vi "Test_Gui_Settings_With_Tabs.vi"() -> ()   [LabVIEW 2015]
uses:
  controls/GUI_Settings_Tabs.ctl
  controls/QMH_Pirenea_MessageCluster.ctl
panel:
  out "error out":errorcluster
  in  "error in (no error)":errorcluster
  in  "Stop":bool
  in  "Start":bool
  in  "Save":bool
  in  "Load":bool
  in  "Exit":bool
  in  "Settings":bool
  out "Commande onglets":enum32{"General", "Hardware", "Experiment"}(tab)
  out "PIL Status":string
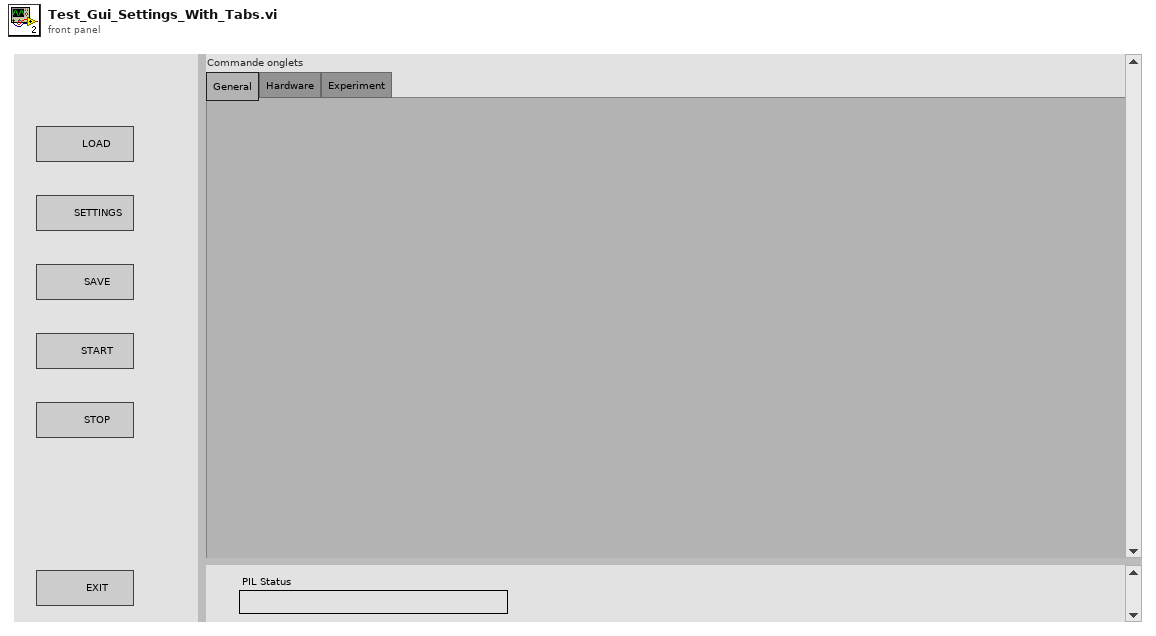
[diagram p1: front panel]
types:
  T1 = enum16{"Initialize", "Load", "Settings", "Save", "Start", "Stop", "Exit"}
  T2 = typedef "QMH_Pirenea_MessageCluster.ctl" = cluster{"Command":enum16{"Initialize", "Load", "Settings", "Save", "Start", "Stop", "Exit"}, "Data":variant}
  T3 = typedef "GUI_Settings_Tabs.ctl" = enum32{"General", "Hardware", "Experiment"}
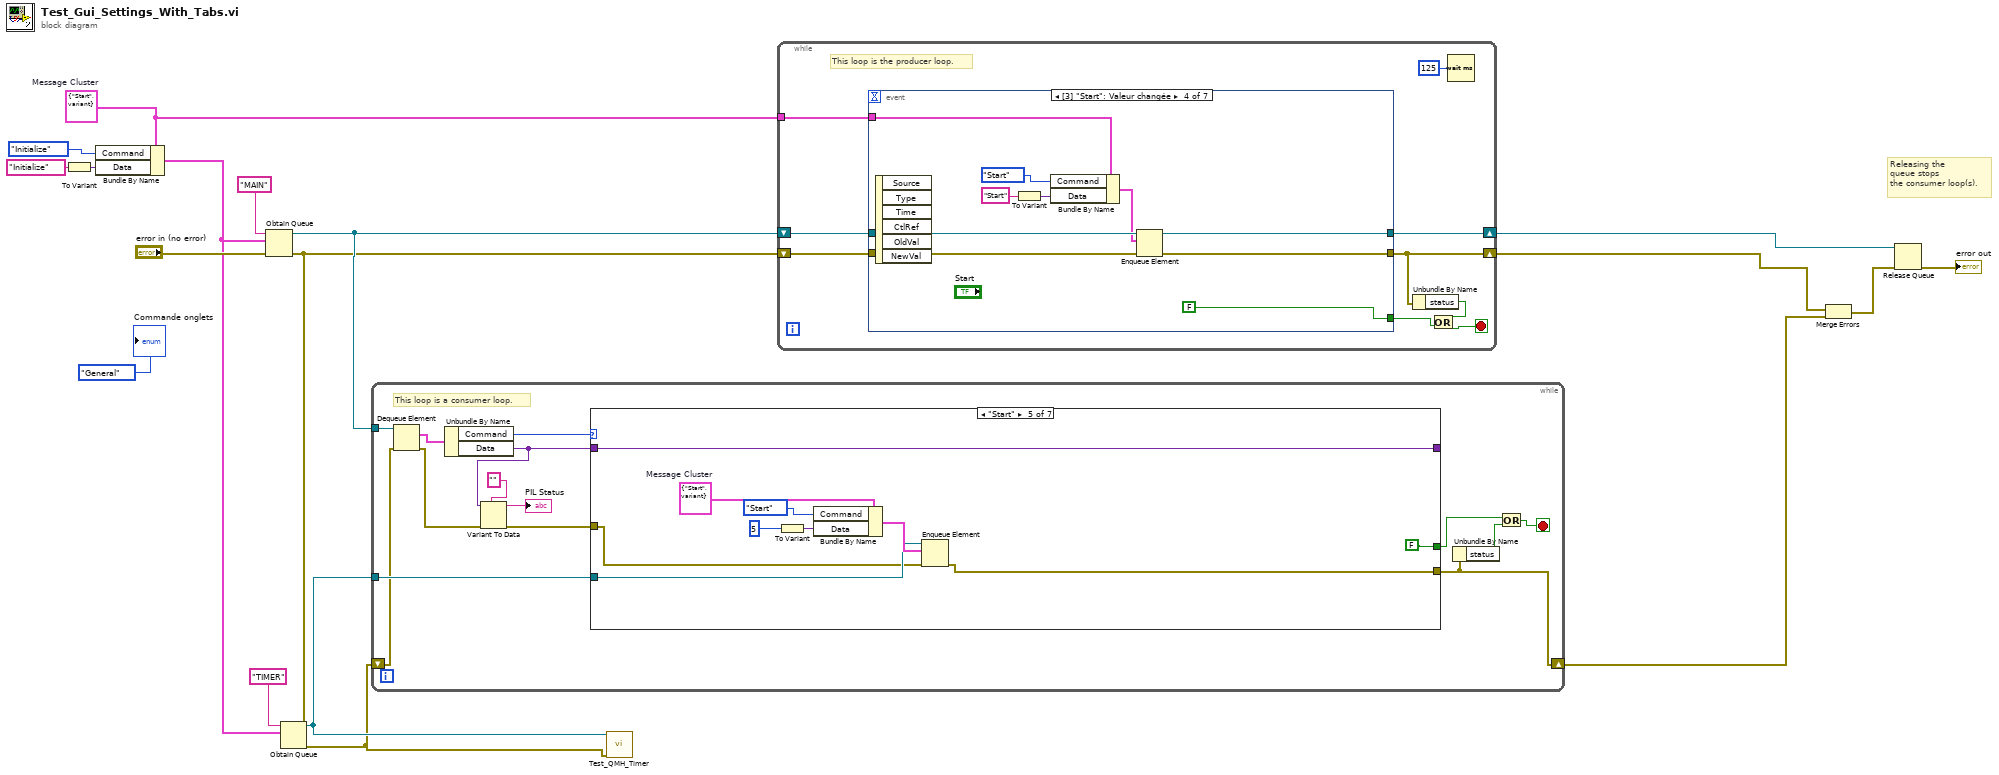
[diagram p0: block diagram]
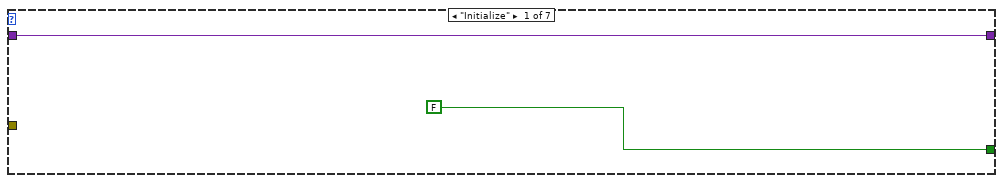
[diagram p2: hidden frame]
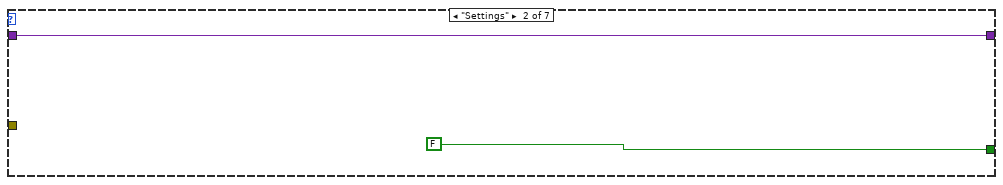
[diagram p3: hidden frame]
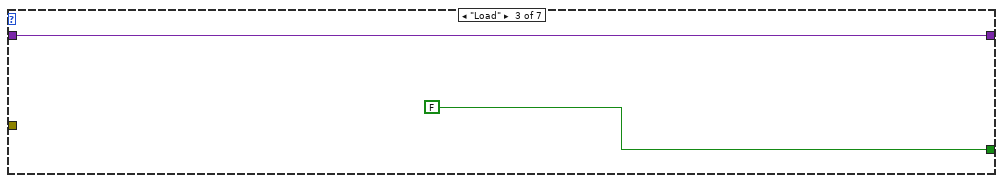
[diagram p4: hidden frame]
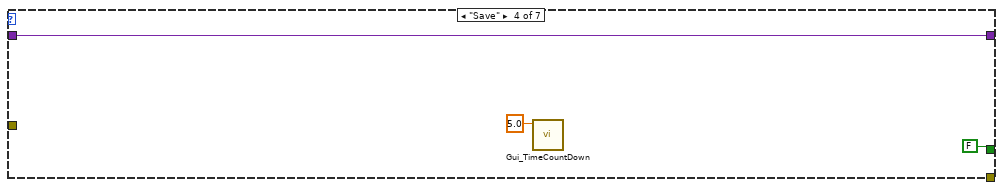
[diagram p5: hidden frame]
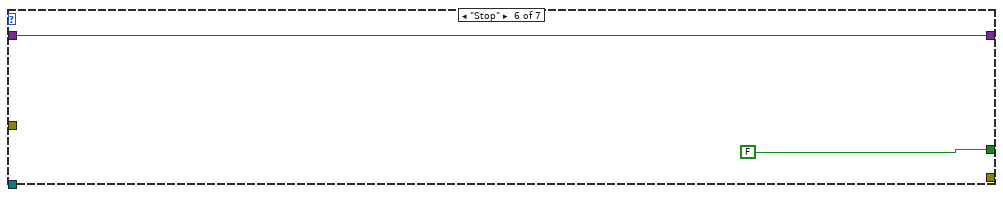
[diagram p6: hidden frame]
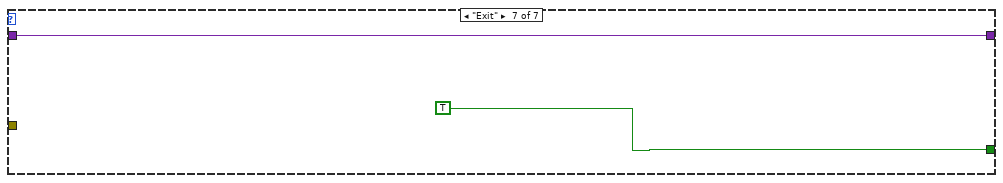
[diagram p7: hidden frame]
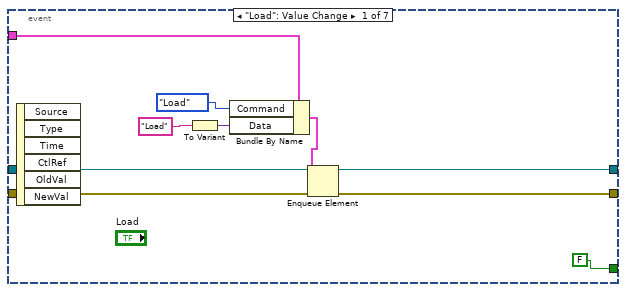
[diagram p8: hidden frame]
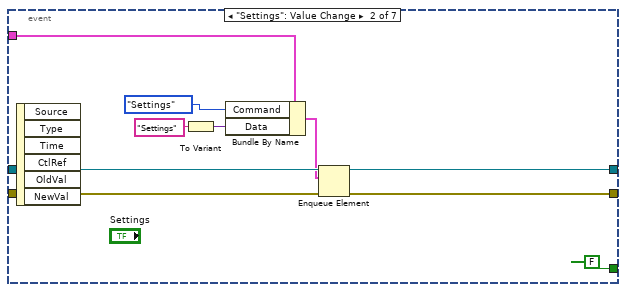
[diagram p9: hidden frame]
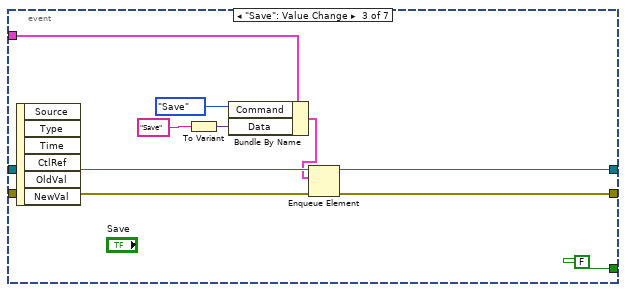
[diagram p10: hidden frame]
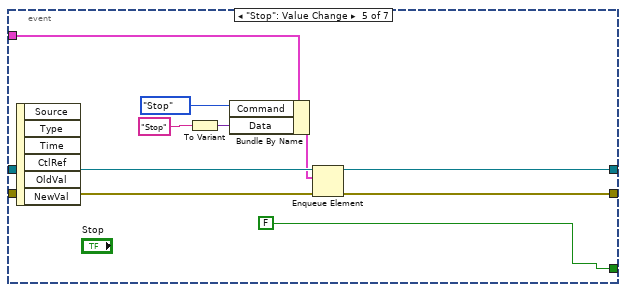
[diagram p11: hidden frame]
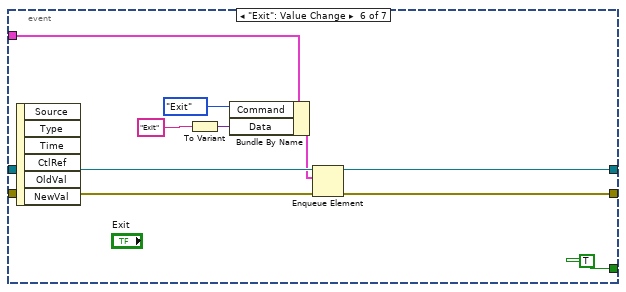
[diagram p12: hidden frame]
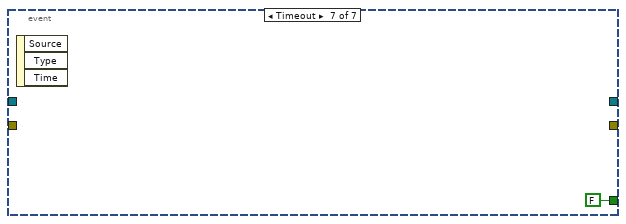
[diagram p13: hidden frame]
diagram:
  w9 = T2 {"Command"=enum."Start", "Data"=variant}  # Message Cluster
  # "Releasing the\nqueue stops\nthe consumer loop(s)."
  n1 = To Variant(anything="Initialize") -> (Variant=w10:variant)
  n2 = Bundle By Name(cluster=w9, "Command"=T1."Initialize", "Data"=w10) -> (w5:T2)
  n3 = Obtain Queue(name (unnamed)="MAIN" ("nom (aucun)"), element data type=w5, error in (no error)="error in (no error)") -> (queue out=w17:refnum<queue>, error out=w4:errorcluster)  [unwired: 2 in, 1 out]
  n4 = Obtain Queue(name (unnamed)="TIMER" ("nom (aucun)"), element data type=w5, error in (no error)=w4) -> (queue out=w2:refnum<queue>, error out=w1:errorcluster)  [unwired: 2 in, 1 out]
  n5 = while {
    tunnel: w17 -> [w31]
    tunnel: w2 -> [w21]
    shift-right: [w19] -> w3
    shift-left: w1 -> [w20]
    stop <- w25 stop-if-true
    # "This loop is a consumer loop."
    n6 = Dequeue Element(queue=w31, error in (no error)=w20) -> (element=w27:T2, error out=w28:errorcluster)  [unwired: 3 out]
    n7 = Unbundle By Name(w27) -> ("Command"=w23:T1, "Data"=w24:variant)
    n8 = Variant To Data(type="", Variant=w24) -> (data=→"PIL Status":string)  [unwired: 1 in, 1 out]
    n9 = case shown="\"Start\"" w23 {
      tunnel: [w32 w34 w36 w40 w49 w51 w53] -> _
      tunnel: [FALSE ("x") FALSE ("x") FALSE ("x") FALSE ("x") FALSE ("x") FALSE ("x") TRUE ("x")] -> w29
      tunnel: w24 -> [w32 w34 w36 w40 w49 w51 w53]
      tunnel: w28 -> [_ _ _ _ w42 _ _]
      tunnel: w21 -> [_ _ _ _ w45 _ _]
      tunnel: [_ _ _ _ w43 _ _] -> w19
      frame "Initialize" {
      }
      frame "Settings" {
      }
      frame "Load" {
      }
      frame "Save" {
        n10 = call "Gui_TimeCountDown.vi"("Seconds"=5.0) -> ()  [unwired: 11 in]
      }
      frame "Start" {
        w44 = T2 {"Command"=enum."Start", "Data"=variant}  # Message Cluster
        n11 = To Variant(anything=5) -> (Variant=w48:variant)
        n12 = Bundle By Name(cluster=w44, "Command"=T1."Start", "Data"=w48) -> (w46:T2)
        n13 = Enqueue Element(queue=w45, element=w46, error in (no error)=w42) -> (error out=w43:errorcluster)  [unwired: 3 out]
      }
      frame "Stop" {
      }
      frame "Exit" {
      }
    }
    n14 = Unbundle By Name(w19) -> ("status"=w30:bool)
    n15 = Or(x=w29, y=w30) -> (x .or. y?=w25:bool)
  }
  n16 = call "Test_QMH_Timer.vi"("error in (no error)"=w1, "Queue TIMER"=w2) -> ()  [unwired: 9 in, 1 out]
  n17 = while {
    shift-right: [w59] -> w12
    shift-left: w4 -> [w60]
    shift-right: [w58] -> w16
    shift-left: w17 -> [w61]
    tunnel: w9 -> [w56]
    stop <- w63 stop-if-true
    # "This loop is the producer loop."
    n18 = event shown="[3] \"Start\": Valeur changée" {
      selector: _ -> [_ _ _ _ _ _ _]
      dyn-events: _ -> [_ _ _ _ _ _ _]
      timeout: _ -> [_ _ _ _ _ _ _]
      tunnel: w61 -> [w73 w83 w93 w103 w113 w123 _]
      tunnel: w60 -> [w72 w82 w92 w102 w112 w122 _]
      tunnel: [w71 w81 w91 w101 w111 w121 _] -> w59
      tunnel: [w70 w80 w90 w100 w110 w120 _] -> w58
      tunnel: [FALSE ("Stop") FALSE ("Stop") FALSE ("Stop") FALSE ("Stop") FALSE ("Stop") TRUE ("Stop") FALSE ("Stop")] -> w57
      tunnel: w56 -> [w66 w76 w86 w96 w106 w116 _]
      event "Load": Value Change {
        n19 = event-data() -> ()  [unwired: 7 out]
        n20 = To Variant(anything="Load") -> (Variant=w68:variant)
        n21 = Bundle By Name(cluster=w66, "Command"=T1."Load", "Data"=w68) -> (w65:T2)
        n22 = Enqueue Element(queue=w73, element=w65, error in (no error)=w72) -> (queue out=w70:refnum<queue>, error out=w71:errorcluster)  [unwired: 2 out]
      }
      event "Settings": Value Change {
        n23 = event-data() -> ()  [unwired: 7 out]
        n24 = To Variant(anything="Settings") -> (Variant=w78:variant)
        n25 = Bundle By Name(cluster=w76, "Command"=T1."Settings", "Data"=w78) -> (w75:T2)
        n26 = Enqueue Element(queue=w83, element=w75, error in (no error)=w82) -> (queue out=w80:refnum<queue>, error out=w81:errorcluster)  [unwired: 2 out]
      }
      event "Save": Value Change {
        n27 = event-data() -> ()  [unwired: 7 out]
        n28 = To Variant(anything="Save") -> (Variant=w88:variant)
        n29 = Bundle By Name(cluster=w86, "Command"=T1."Save", "Data"=w88) -> (w85:T2)
        n30 = Enqueue Element(queue=w93, element=w85, error in (no error)=w92) -> (queue out=w90:refnum<queue>, error out=w91:errorcluster)  [unwired: 2 out]
      }
      event "Start": Value Change {
        n31 = event-data() -> ()  [unwired: 7 out]
        n32 = To Variant(anything="Start") -> (Variant=w97:variant)
        n33 = Bundle By Name(cluster=w96, "Command"=T1."Start", "Data"=w97) -> (w95:T2)
        n34 = Enqueue Element(queue=w103, element=w95, error in (no error)=w102) -> (queue out=w100:refnum<queue>, error out=w101:errorcluster)  [unwired: 2 out]
      }
      event "Stop": Value Change {
        n35 = event-data() -> ()  [unwired: 7 out]
        n36 = To Variant(anything="Stop") -> (Variant=w108:variant)
        n37 = Bundle By Name(cluster=w106, "Command"=T1."Stop", "Data"=w108) -> (w105:T2)
        n38 = Enqueue Element(queue=w113, element=w105, error in (no error)=w112) -> (queue out=w110:refnum<queue>, error out=w111:errorcluster)  [unwired: 2 out]
      }
      event "Exit": Value Change {
        n39 = event-data() -> ()  [unwired: 7 out]
        n40 = To Variant(anything="Exit") -> (Variant=w118:variant)
        n41 = Bundle By Name(cluster=w116, "Command"=T1."Exit", "Data"=w118) -> (w115:T2)
        n42 = Enqueue Element(queue=w123, element=w115, error in (no error)=w122) -> (queue out=w120:refnum<queue>, error out=w121:errorcluster)  [unwired: 2 out]
      }
      event Timeout {
        n43 = event-data() -> ()  [unwired: 4 out]
      }
    }
    n44 = Unbundle By Name(w59) -> ("status"=w62:bool)
    n45 = Or(x=w62, y=w57) -> (x .or. y?=w63:bool)
    n46 = Wait (ms)(milliseconds to wait=u32 125) -> ()  [unwired: 1 out]
  }
  n47 = Merge Errors(w12, w3) -> (w13:errorcluster)
  n48 = Release Queue(queue=w16, error in (no error)=w13) -> (error out=→"error out":errorcluster)  [unwired: 3 out]
  "Commande onglets" <- GUI_Settings_Tabs."General" ("Commande onglets")
